vi "000 Aleatori shift register 2.vi"() -> ()   [LabVIEW 2019]
uses:
  <vilib>/numeric/Random Number (Range) DBL.vi
panel:
  in  "Divisor 2":dbl
  out "Número Aleatori 2":dbl
  out "Resultat 2":dbl format="%#_4g"
  in  "Genera nombre aleatori\nEntre 5 i 25":bool
  in  "stop 2":bool
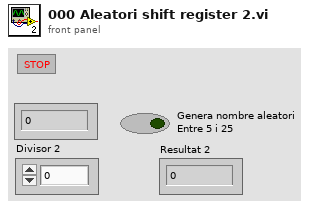
[diagram p1: front panel]
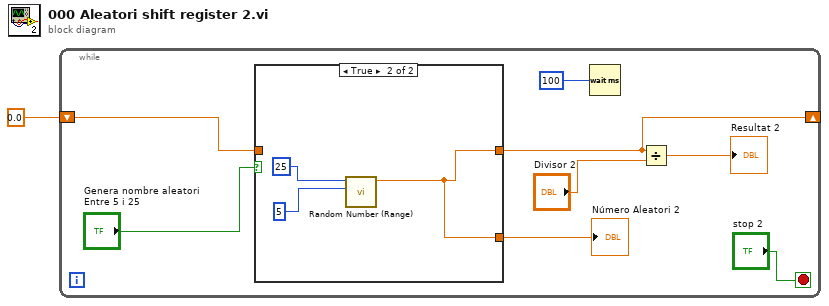
[diagram p0: block diagram]
diagram:
  n1 = while {
    shift-right: [w5] -> _
    shift-left: 0.0 -> [w4]
    stop <- "stop 2" stop-if-true
    n2 = case shown="True" "Genera nombre aleatori\nEntre 5 i 25" {
      tunnel: [w10 w11] -> w6
      tunnel: [w10 w11] -> w5
      tunnel: w4 -> [w10 _]
      frame False {
      }
      frame True {
        n3 = call-poly <vilib>:"Random Number (Range).vi"("lower bound (0)"=5, "upper bound (100)"=25) -> ("number"=w11:dbl)  [unwired: 9 in]
      }
    }
    "Número Aleatori 2" <- w6
    n4 = Wait (ms)(milliseconds to wait=100) -> ()  [unwired: 1 out]
    n5 = Divide(x=w5, y="Divisor 2") -> (x/y=→"Resultat 2":dbl)
  }
